vi "create_save_folder-v02.vi"(8 "error in (no error)":errorcluster, 9 "which manipulator":T1(ring), 10 "current cell":i32, 11 "log path":path) -> (0 "error out":errorcluster, 1 "Recording":string, 2 "Date":string, 3 "dup path":path)   [LabVIEW 2015]
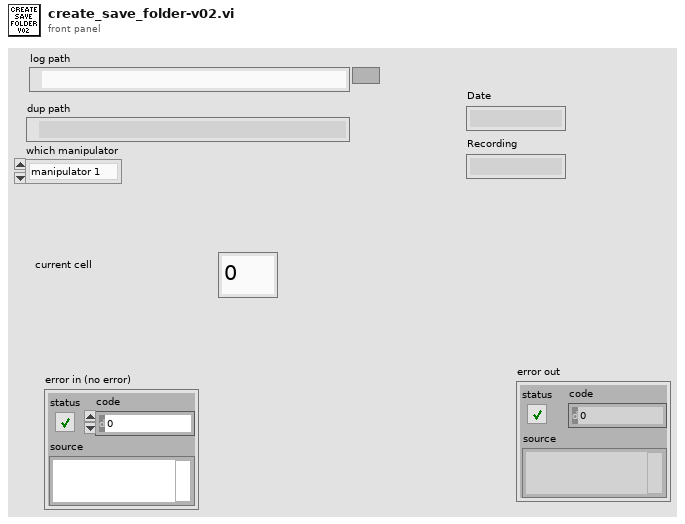
[diagram p1: front panel]
types:
  T1 = enum16{"manipulator 1", "manipulator 2", "manipulator 3", "manipulator 4"}
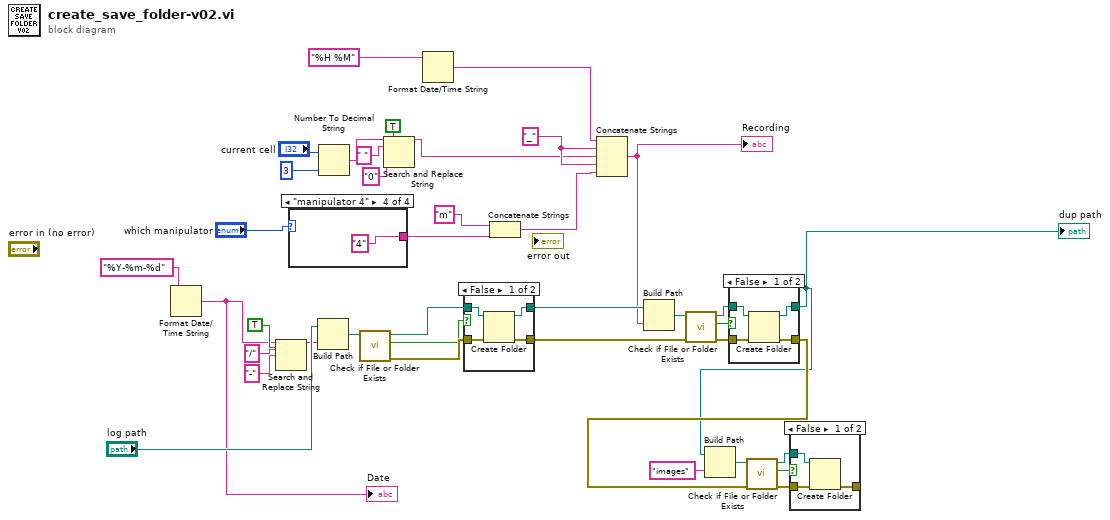
[diagram p0: block diagram]
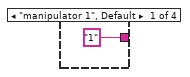
[diagram p3: hidden frame]
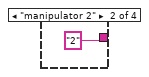
[diagram p4: hidden frame]
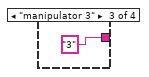
[diagram p5: hidden frame]
diagram:
  w24 = "_" ("string")
  n1 = Format Date/Time String(time format string (%c)="%Y-%m-%d") -> (date/time string=w3:string)  [unwired: 2 in]
  "Date" <- w3
  n2 = Search and Replace String(replace all?=TRUE ("replace all? (F)"), input string=w3, search string="/", replace string="-" ("replace string (\"\")")) -> (result string=w27:string)  [unwired: 4 in, 3 out]
  n3 = case shown="\"manipulator 4\"" "which manipulator" {
    tunnel: ["1" "2" "3" "4"] -> w21
    frame "manipulator 1", Default {
    }
    frame "manipulator 2" {
    }
    frame "manipulator 3" {
    }
    frame "manipulator 4" {
    }
  }
  n4 = Build Path(base path="log path", name or relative path=w27) -> (appended path=w31:path)
  n5 = Number To Decimal String(number="current cell", width (-)=3) -> (decimal integer string=w16:string)
  n6 = call <vilib>:"Check if File or Folder Exists.vi"("path"=w31) -> ("error out"=w32:errorcluster, "file or folder exists?"=w30:bool, "dup path"=w33:path)  [unwired: 8 in]
  n7 = Search and Replace String(replace all?=TRUE, input string=w16, search string=" ", replace string="0") -> (result string=w2:string)  [unwired: 4 in, 3 out]
  n8 = Format Date/Time String(time format string (%c)="%H %M") -> (date/time string=w17:string)  [unwired: 2 in]
  n9 = case shown="False" w30 {
    tunnel: [w47 w49] -> w28
    tunnel: [w46 w48] -> w35
    tunnel: w32 -> [w45 w48]
    tunnel: w33 -> [w44 w49]
    frame False {
      n10 = Create Folder(path (use dialog)=w44, error in=w45) -> (created path=w47:path, error out=w46:errorcluster)  [unwired: 1 in, 1 out]
    }
    frame True {
    }
  }
  n11 = Concatenate Strings("m", w21) -> (w19:string)
  n12 = Concatenate Strings(w17, w24, w2, w24, w19) -> (w1:string)
  "Recording" <- w1
  n13 = Build Path(base path=w28, name or relative path=w1) -> (appended path=w34:path)
  n14 = call <vilib>:"Check if File or Folder Exists.vi"("error in (no error)"=w35, "path"=w34) -> ("error out"=w37:errorcluster, "file or folder exists?"=w36:bool, "dup path"=w38:path)  [unwired: 7 in]
  n15 = case shown="False" w36 {
    tunnel: [w53 w55] -> w5
    tunnel: [w52 w54] -> w6
    tunnel: w37 -> [w51 w54]
    tunnel: w38 -> [w50 w55]
    frame False {
      n16 = Create Folder(path (use dialog)=w50, error in=w51) -> (created path=w53:path, error out=w52:errorcluster)  [unwired: 1 in, 1 out]
    }
    frame True {
    }
  }
  "dup path" <- w5
  n17 = Build Path(base path=w5, name or relative path="images") -> (appended path=w7:path)
  n18 = call <vilib>:"Check if File or Folder Exists.vi"("error in (no error)"=w6, "path"=w7) -> ("error out"=w9:errorcluster, "file or folder exists?"=w8:bool, "dup path"=w10:path)  [unwired: 7 in]
  n19 = case shown="False" w8 {
    tunnel: [w58 w59] -> _
    tunnel: w9 -> [w57 w59]
    tunnel: w10 -> [w56 _]
    frame False {
      n20 = Create Folder(path (use dialog)=w56, error in=w57) -> (error out=w58:errorcluster)  [unwired: 1 in, 2 out]
    }
    frame True {
    }
  }
